vi "NotificationBar.vi"(9 "NotificationBarString":string) -> ()   [LabVIEW 2012]
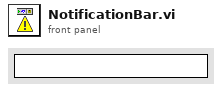
[diagram p1: front panel]
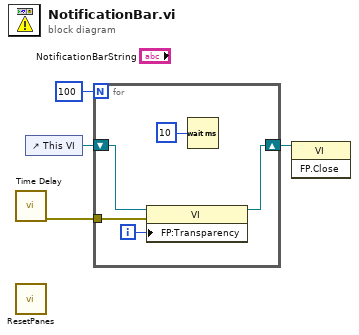
[diagram p0: block diagram]
diagram:
  n1 = call "Time Delay"() -> ("error out"=w2:errorcluster)  [unwired: 11 in]
  n2 = call "ResetPanes.vi"() -> ()  [unwired: 12 in]
  n3 = control-ref of="This VI"() -> (w1:refnum<vi>)
  n4 = for {
    N: 100 -> [_]
    tunnel: w2 -> [w6]
    shift-right: [w5] -> w3
    shift-left: w1 -> [w9]
    i -> [w8]
    n5 = property class="VI"(reference=w9, error in=w6, "FP:Transparency"=w8) -> (reference out=w5:refnum<vi>)  [unwired: 1 out]
    n6 = Wait (ms)(milliseconds to wait=u32 10) -> ()  [unwired: 1 out]
  }
  n7 = invoke class="VI" method="FP.Close"(reference=w3) -> ()  [unwired: 2 in, 3 out]
